vi "Configure Active Compliance.vi"(8 "error in (no error)":errorcluster, 9 "Active Compliance Settings":T1={"Clockwise Slope (9.38416 deg)"=9.384164, "Counter-Clockwise Slope (9.38416 deg)"=9.384164, "Clockwise Margin (0.293255 deg)"=0.29325512, "Counter-Clockwise Margin (0.293255 deg)"=0.29325512, "Punch (3.12805%)"=3.12805, "Max  Torque (100%)"=100.0}, 10 "Motor ID (0)":u8, 11 "Dynamixel Motor in":refnum<class "Dynamixel Motor.lvclass">) -> (0 "error out":errorcluster, 3 "Dynamixel Motor out":refnum<class "Dynamixel Motor.lvclass">)   [LabVIEW 2016, in "Dynamixel Motor.lvclass"]
doc: "Adjusts the active compliance of the motor. See the motor's user manual for more details."
uses:
  <instrlib>/Dynamixel Motor/HAIOL/Dynamixel Motor.lvclass
  <instrlib>/Dynamixel Motor/Public/Configure/Active Compliance Settings.ctl
  <instrlib>/Dynamixel Motor/Dynamixel Motor.lvlib
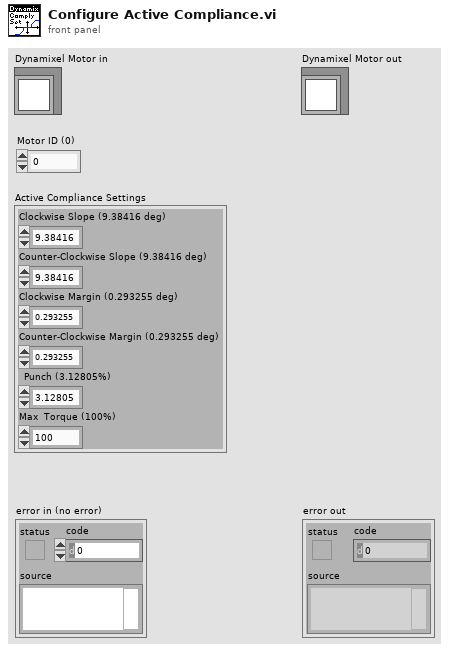
[diagram p1: front panel]
types:
  T1 = typedef "Dynamixel Motor.lvlib/Active Compliance Settings.ctl" = cluster{"Clockwise Slope (9.38416 deg)":sgl, "Counter-Clockwise Slope (9.38416 deg)":sgl, "Clockwise Margin (0.293255 deg)":sgl, "Counter-Clockwise Margin (0.293255 deg)":sgl, "Punch (3.12805%)":sgl, "Max  Torque (100%)":sgl}
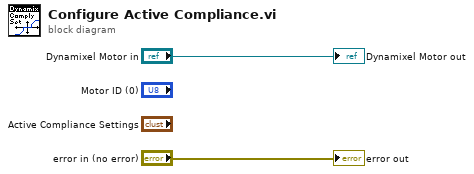
[diagram p0: block diagram]
diagram:
  "error out" <- "error in (no error)"
  "Dynamixel Motor out" <- "Dynamixel Motor in"
